vi "niRFUtil MASMT Decimate (single shot) (CDB).vi"(8 "error in (no error)":errorcluster, 9 "averaging":bool, 10 "decimating factor":i32=1, 11 "X":cdb[](array[numeric])) -> (0 "error out":errorcluster, 3 "Decimated X":cdb[](array[numeric]))   [LabVIEW 2015, in "niRFUtil.lvlib"]
doc: "Decimates the input sequence <B>X</B> by the <B>decimating factor</B>."
uses:
  niRFUtil.lvlib
  Utilities/niRFMASMT_FFT.dll
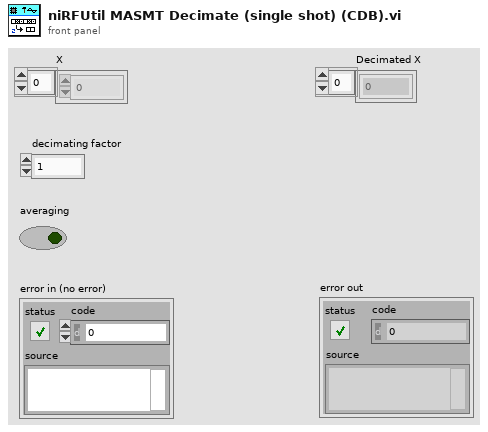
[diagram p1: front panel]
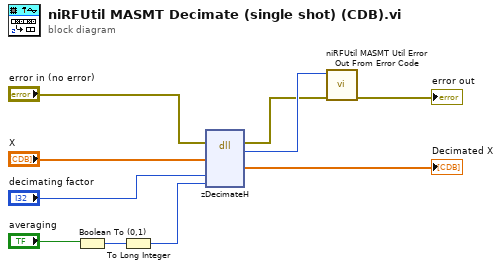
[diagram p0: block diagram]
diagram:
  n1 = Boolean To (0,1)(Boolean="averaging") -> (0, 1=w3:i16)
  n2 = To Long Integer(number=w3) -> (32bit integer=w1:i32)
  n3 = dll-call lib="C:/Perforce/semoore-sales/Customers/NATI-3813/Noise Floor/LV Filters/ParallelComplexFilterRFUtil/niRFUtil/MASMT/Utilities/niRFMASMT_FFT.*" fn="zDecimateH"(error in="error in (no error)", "xH"="X", "factor"="decimating factor", "average"=w1) -> (error out=w4:errorcluster, "return type"=w8:i32, "Decimated X"=→"Decimated X":cdb[])  [unwired: 6 in, 1 out]
  n4 = call "niRFUtil MASMT Util Error Out From Error Code.vi"("error in (no error)"=w4, "error code"=w8) -> ("error out"=→"error out":errorcluster)  [unwired: 9 in]
